vi "Sodium Boiler Model.vi"(5 "Heated Coolant Input (mB/t)":i64, 7 "Superheating Elements":i32=3 min=1 max=63 step=1, 8 "Steam Cavity Height (m)":i32, 9 "Water Cavity Height (m)":i32, 10 "Length (m)":i32=3 min=3 max=18 step=1, 11 "Width (m)":i32=4 min=3 max=18 step=1) -> (4 "Boiler Build Properties":T1={"Water Tank (mB)"=0, "Steam Tank (mB)"=0, "Heated Coolant Tank (mB)"=0, "Coolant Tank (mB)"=0, "Maximum Boil Rate (mB/t)"=4, "Height (m)"=4, "Volume (m³)"=0} {"Height (m)" min=4 max=18 step=1; "Maximum Boil Rate (mB/t)" min=4 max=18 step=1})   [LabVIEW 2023]
uses:
  Boiler Build Properties.ctl
panel:
  out "Steam Tubes Required":u32=4 min=4 max=18 step=1
  out "Status":bool
  out "Water Demand (mB/t)":i64
  out "Boil Rate (mB/t)":dbl(slide) scale=0.0..2240000.0 scale format="%#_6f"
  out "Sodium Loops Required":u32=4 min=4 max=18 step=1
  out "Water Pipes Required":u32=4 min=4 max=18 step=1
  out "Steam Output (mB/t)":i64
  out "Coolant Output (mB/t)":i64
  out "Pressure Dispersers":i32=4 min=4 max=18 step=1
  # "Thermoelectric Boiler Properties"
  # "Note: The boiler's heated coolant tank size must be about twice the size of the\nreactor's coolant tank, with as much coolant buffered in the coolant return tube\nand as much water as the water tank's capacity buffered in the water return tubes."
  # "Thermoelectric Boiler Operation"
  # "+1 for heating elements"
  # "+1 for dispersers"
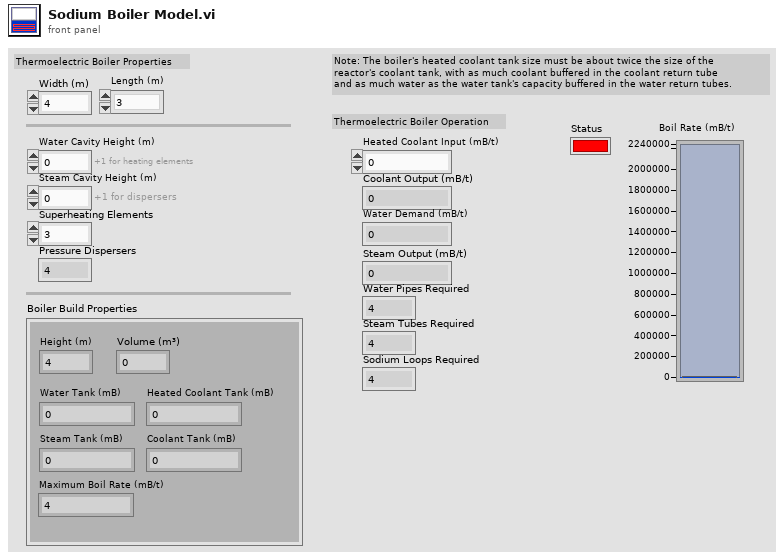
[diagram p1: front panel]
types:
  T1 = typedef "Boiler Build Properties.ctl" = cluster{"Water Tank (mB)":i32, "Steam Tank (mB)":i32, "Heated Coolant Tank (mB)":i64, "Coolant Tank (mB)":i64, "Maximum Boil Rate (mB/t)":i32, "Height (m)":i32, "Volume (m³)":i32}
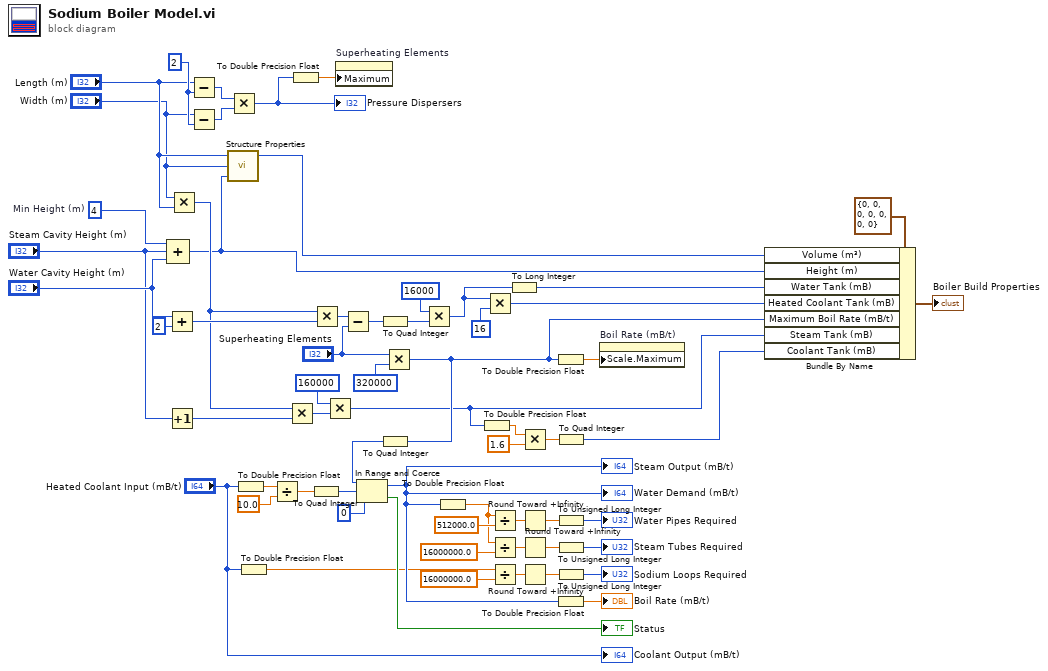
[diagram p0: block diagram]
diagram:
  w55 = 2 ("y")
  w61 = 4  # Min Height (m)
  n1 = Compound Arithmetic op=ADD(w61, "Steam Cavity Height (m)", "Water Cavity Height (m)") -> (w2:i32)
  n2 = Add(x="Water Cavity Height (m)", y=2) -> (x+y=w44:i32)
  n3 = Increment(x="Steam Cavity Height (m)") -> (x+1=w42:i32)
  n4 = Multiply(x="Width (m)", y="Length (m)") -> (x*y=w43:i32)
  n5 = Subtract(x="Length (m)", y=w55) -> (x-y=w54:i32)
  n6 = Subtract(x="Width (m)", y=w55) -> (x-y=w53:i32)
  n7 = call "Structure Properties.vi"("Length"="Length (m)", "Width"="Width (m)", "Height"=w2) -> ("Volume"=w3:i32)  [unwired: 2 in, 4 out]
  n8 = Multiply(x=w54, y=w53) -> (x*y=w15:i32)
  "Pressure Dispersers" <- w15
  n9 = To Double Precision Float(number="Heated Coolant Input (mB/t)") -> (double precision float=w30:dbl)
  n10 = To Double Precision Float(number="Heated Coolant Input (mB/t)") -> (double precision float=w22:dbl)
  n11 = Divide(x=w30, y=10.0) -> (x/y=w31:dbl)
  n12 = Multiply(x=w43, y=w42) -> (x*y=w48:i32)
  n13 = To Double Precision Float(number=w15) -> (double precision float=w14:dbl)
  n14 = To Quad Integer(1:w31) -> (0:w28:i64)
  n15 = Multiply(x=w43, y=w44) -> (x*y=w58:i32)
  n16 = Multiply(x=160000 ("y"), y=w48) -> (x*y=w4:i32)
  n17 = property on="Superheating Elements" class="DigNum (strict)"("Maximum"=w14) -> ()  [unwired: 2 in, 2 out]
  n18 = Subtract(x=w58, y="Superheating Elements") -> (x-y=w56:i32)
  n19 = To Quad Integer(1:w56) -> (0:w11:i64)
  n20 = Multiply(x="Superheating Elements", y=320000) -> (x*y=w5:i32)
  n21 = To Quad Integer(1:w5) -> (0:w10:i64)
  n22 = In Range and Coerce(upper limit=w10, x=w28, lower limit=i64 0) -> (coerced(x)=w24:i64, In Range?=→"Status":bool)
  "Steam Output (mB/t)" <- w24
  "Water Demand (mB/t)" <- w24
  n23 = Multiply(x=i64 16000 ("y"), y=w11) -> (x*y=w52:i64)
  n24 = To Double Precision Float(number=w24) -> (double precision float=w16:dbl)
  n25 = To Double Precision Float(number=w4) -> (double precision float=w26:dbl)
  n26 = Multiply(x=w52, y=i64 16) -> (x*y=w6:i64)
  n27 = Divide(x=w16, y=512000.0) -> (x/y=w38:dbl)
  n28 = Divide(x=w16, y=16000000.0) -> (x/y=w18:dbl)
  n29 = Divide(x=w22, y=16000000.0) -> (x/y=w37:dbl)
  n30 = To Long Integer(number=w52) -> (32bit integer=w8:i32)
  n31 = Multiply(x=w26, y=1.6) -> (x*y=w46:dbl)
  n32 = Round Toward +Infinity(x=w38) -> (ceil(x): smallest int >= x=w36:dbl)
  n33 = Round Toward +Infinity(x=w18) -> (ceil(x): smallest int >= x=w19:dbl)
  n34 = Round Toward +Infinity(x=w37) -> (ceil(x): smallest int >= x=w35:dbl)
  n35 = To Double Precision Float(number=w5) -> (double precision float=w25:dbl)
  n36 = To Quad Integer(1:w46) -> (0:w1:i64)
  n37 = To Unsigned Long Integer(number=w36) -> (unsigned 32bit integer=→"Water Pipes Required":u32)
  n38 = To Unsigned Long Integer(number=w19) -> (unsigned 32bit integer=→"Steam Tubes Required":u32)
  n39 = To Unsigned Long Integer(number=w35) -> (unsigned 32bit integer=→"Sodium Loops Required":u32)
  n40 = To Double Precision Float(number=w24) -> (double precision float=→"Boil Rate (mB/t)":dbl)
  n41 = property on="Boil Rate (mB/t)" class="Slide (strict)"("Scale.Maximum"=w25) -> ()  [unwired: 2 in, 2 out]
  n42 = Bundle By Name(cluster=T1 {"Water Tank (mB)"=0, "Steam Tank (mB)"=0, "Heated Coolant Tank (mB)"=0, "Coolant Tank (mB)"=0, "Maximum Boil Rate (mB/t)"=0, "Height (m)"=0, "Volume (m³)"=0} ("Boiler Build Properties"), "Volume (m³)"=w3, "Height (m)"=w2, "Water Tank (mB)"=w8, "Heated Coolant Tank (mB)"=w6, "Maximum Boil Rate (mB/t)"=w5, "Steam Tank (mB)"=w4, "Coolant Tank (mB)"=w1) -> (→"Boiler Build Properties":T1)
  "Coolant Output (mB/t)" <- "Heated Coolant Input (mB/t)"
